vi "Converting HEX strings to Ascii strings.vi"(11 "chaîne IN":string) -> (2 "Chaine":string[](array[string]), 3 "Chaîne OUT":string)   [LabVIEW 2020, in "Library Commun.lvlib"]
uses:
  Library Commun.lvlib
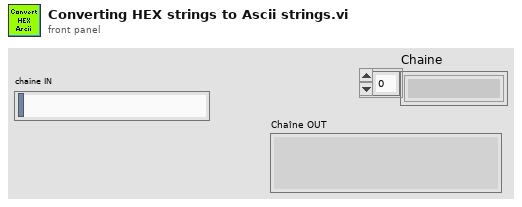
[diagram p1: front panel]
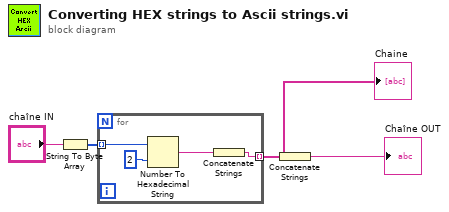
[diagram p0: block diagram]
diagram:
  n1 = String To Byte Array(string="chaîne IN") -> (unsigned byte array=w2:u8[])
  n2 = for {
    tunnel: w2 -> [w8] mode=indexing
    tunnel: [w6] -> w3 mode=indexing
    n3 = Number To Hexadecimal String(1:i16 2 ("largeur (-)"), 2:w8) -> (0:w7:string)
    n4 = Concatenate Strings(w7) -> (w6:string)
  }
  "Chaine" <- w3
  n5 = Concatenate Strings(w3) -> (→"Chaîne OUT":string)
